vi "Dummy functional data generator.vi"() -> ()   [LabVIEW 2020]
uses:
  User Interface/Visualisation/Functional Imaging Viewer/SubVIs/Experiment header interface/Typedefs/Header file interface module functions enum.ctl
  Typedefs/Imaging Protocols enum.ctl
  Typedefs/Logging queue element.ctl
  Typedefs/Frame Size.ctl
  Typedefs/Acquired points count.ctl
panel:
  in  "Array":T1[](array[typedef]) {"Ref Dwell time (us)" format="%#.6g"; "Frame Size" items=["100X100"=100, "128X128"=128, "200X200"=200, "256X256"=256, "512X512"=512, "1024x1024"=1024, "2048x2048"=2048]; "Dwell time (us)" format="%#.6g"}
  out "error out":errorcluster
  in  "File path of existing dataset":path=path "C:/Functional Imaging Code/Data_Dummy generated -1POI 1Mscn"
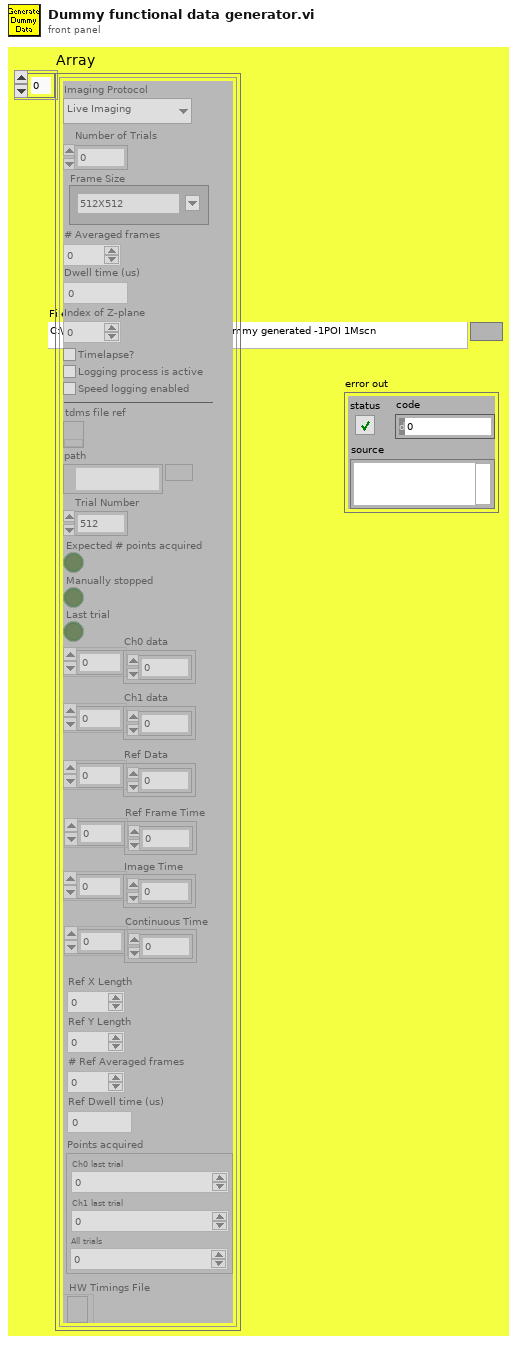
[diagram p1: front panel]
types:
  T1 = typedef "Logging queue element.ctl" = cluster{"Imaging Protocol":T2, "Number of Trials":u16, "Frame Size":T3, "# Averaged frames":u16, "Dwell time (us)":dbl, "Index of Z-plane":i32, "Timelapse?":bool, "Logging process is active":bool, "Speed logging enabled":bool, "tdms file ref":refnum<k34>, "path":path, "Trial Number":i32, "Expected # points acquired":bool, "Manually stopped":bool, "Last trial":bool, "Ch0 data":u32[], "Ch1 data":u32[], "Ref Data":u32[], "Ref Frame Time":u64[], "Image Time":u64[], "Continuous Time":u64[], "Ref X Length":u16, "Ref Y Length":u16, "# Ref Averaged frames":u16, "Ref Dwell time (us)":dbl, "Points acquired":T4, "HW Timings File":refnum<file>}
  T2 = typedef "Imaging Protocols enum.ctl" = enum16{"AOL Z-Stack", "Motor Z Stack", "Functional Acquisition", "Single Plane Acquisition", "Volume Acquisition", "Live Imaging", "Live Plane Imaging", "Live Volume Imaging"}
  T3 = typedef "Frame Size.ctl" = u16
  T4 = typedef "Acquired points count.ctl" = cluster{"Ch0 last trial":u64, "Ch1 last trial":u64, "All trials":u64}
  T5 = typedef "Header file interface module functions enum.ctl" = enum16{"Load experiment header file", "Save experiment header file", "Clear stored values", "Read stored values", "Update specific value in memory", "Update values in memory"}
  T6 = typedef "Header parameters cluster-ALL.ctl" = cluster{"LOGIN":T7, "GLOBAL PARAMETERS":T8, "IMAGING MODES":T10, "TIME SERIES":T11, "MOTOR Z-STACK ":T13, "AOL Z-STACK":T14, "FUNCTIONAL IMAGING":T15, "VOLUME IMAGING":T15, "MOVEMENT CORRECTION":T19, "CALIBRATION":T21, "STATISTICS":T22, "BIOLOGY INFORMATION":T23, "Calibration Data":T24}
  T7 = typedef "Header params -Login.ctl" = cluster{"User":string, "Profile":string, "Software Version":string, "Experiment Date Time":timestamp}
  T8 = typedef "Header params-Global Parameters.ctl" = cluster{"MicroscopeID":string, "Microscope Type":string, "Objective":string, "Field of View (um)":dbl, "Fill time (us)":dbl, "Experiment Type":T9, "Stimuli Trigger":bool, "Speed Logging":bool}
  T9 = typedef "Experiment Type.ctl" = enum16{"In vivo", "In vitro", "Testing", "Calibration", "Other"}
  T10 = typedef "Header params-Imaging Modes.ctl" = cluster{"Time Series":bool, "Motor Zstack":bool, "AOL Zstack":bool, "Functional Imaging":bool, "Volume Imaging":bool}
  T11 = typedef "Header params-Time Series.ctl" = cluster{"Basic Image meta data":T12, "AOL z":dbl}
  T12 = typedef "Header params-Basic image meta data.ctl" = cluster{"Wavelength (nm)":dbl, "# averaged frames":dbl, "laser power (%)":dbl, "Pockels":dbl, "pixel dwell time (us)":dbl, "pmt 1":dbl, "pmt 2":dbl, "back apperture":dbl, "zoom":dbl, "field of view":dbl, "Frame Size":T3, "AOL x centre":dbl, "AOL y centre":dbl, "Stage x position":dbl, "Stage y position":dbl, "Stage z position":dbl}
  T13 = typedef "Header params-Motor Z-stack.ctl" = cluster{"Hdr Basic Image meta data":T12, "Z Start":dbl, "Z Stop":dbl, "No of Planes":i32, "Laser Power (%) at Z Start":dbl, "Laser Power (%) at Z Stop":dbl}
  T14 = typedef "Header params-AOL Z-stack.ctl" = cluster{"Hdr Basic Image meta data":T12, "Z Start":dbl, "Z Stop":dbl, "No of Planes":i32, "Laser Power (%) at Z Start":dbl, "Laser Power (%) at Z Stop":dbl}
  T15 = typedef "Header params-Functional Imaging.ctl" = cluster{"Functional Mode":T16, "Variable Length":bool, "Variable Resolution":bool, "Pockels Modulation":bool, "Stimuli Trigger":bool, "Cool down enabled":bool, "AOL Mode":T17, "Plane Mode":T18, "Miniscan Dwell time per pixel (us)":dbl, "poi dwell time":dbl, "Number of trials":dbl, "Number of cycles":dbl, "Number of pois":dbl, "Number of miniscans":dbl, "Number of pixels in miniscan":dbl, "Rectangle ROI length":dbl, "Rectangle ROI height":dbl, "Frame rate (fps)":dbl, "Acquisition Length":dbl, "video length (sec)":dbl, "Stimuli delay (sec)":dbl, "Cool down time (sec)":dbl, "Basic Image meta data":T12, "Z Start (um)":dbl, "Z Stop (um)":dbl}
  T16 = typedef "Functional Mode.ctl" = enum16{"Point", "Line", "Patch", "Plane", "Volume"}
  T17 = typedef "AOL modes.ctl" = enum16{"Raster", "Structural", "Pointing", "Mini Scan", "Alignment"}
  T18 = typedef "Plane Mode.ctl" = u16
  T19 = typedef "Header params-Movement correction.ctl" = cluster{"Movement Correction":bool, "Axial Reference":bool, "Reference Source":T20, "Full Frame Size":dbl, "Reference Field of View":dbl, "Reference Zoom":dbl, "Reference dwell time (us)":dbl, "Reference X Pixels":dbl, "Reference Y Pixels":dbl, "Number of Z lines":dbl, "Size of Z pixels":dbl, "Axial Pixels":dbl, "Ignore Z lines":dbl, "Reference Scan Cycles":dbl, "Reference Threshold XY":dbl, "Reference Threshold Z":dbl, "Reference Average XY":dbl, "Reference Average Z":dbl, "Proportional Scale":dbl, "Integral Scale":dbl, "Proportional Scale Z":dbl, "Integral Scale Z":dbl, "Diff Threshold":dbl, "Diff Threshold Z":dbl, "Sliding Average":bool, "Reference count reset enabled":bool, "Scan Interval (ms)":dbl, "Ref Plot Refresh Rate (ms)":dbl}
  T20 = typedef "Reference source.ctl" = enum16{"Green channel", "Red channel"}
  T21 = typedef "Header params-Calibration Setup.ctl" = cluster{"Pockels Calibration File":path, "Calibration_ini file":path, "Setup_ini file":path}
  T22 = typedef "Header params-statistics.ctl" = cluster{"Z-stack duration (sec)":dbl, "Number of acquired data-points":dbl, "Acquisition time (ms)":dbl, "Number of acquired frames":dbl, "Intertrial times":dbl[]}
  T23 = typedef "Biology Information.ctl" = cluster{"Animal Code or Name":string, "Animal DoB":string, "Animal Age":string, "Animal Sex":string, "Animal Weight":string, "Date of Injection":string, "Date of Implant":string, "Site of Injection":string, "Animal Ear Notch":string, "AAV constructs":string, "Genetic background":string, "Optical reporter":string, "Region of brain imaged":string, "Other \ncomments":string}
  T24 = typedef "Header params-calibration data.ctl" = cluster{"Objective Name":string, "Calibration Wavelength":dbl, "Sum X":dbl, "Sum Y":dbl, "Diff X":dbl, "Diff Y":dbl, "Distortion Correction":dbl, " Z norm to um Scaling":dbl, " X norm to um Scaling":dbl}
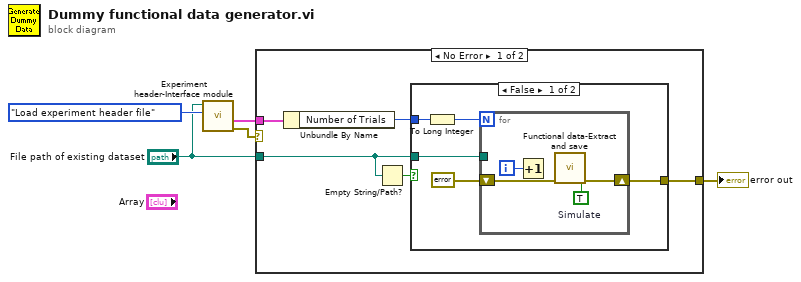
[diagram p0: block diagram]
diagram:
  n1 = call "Experiment header-Interface module.vi"("Function"=Header_file_interface_module_functions_enum."Load experiment header file", "Experiment data folder path"="File path of existing dataset") -> ("error out"=w1:errorcluster, "All header parameters out"=w2:T6)  [unwired: 8 in]
  n2 = case shown="No Error" w1 {
    tunnel: [w10 _] -> w5
    tunnel: "File path of existing dataset" -> [w7 _]
    tunnel: w2 -> [w6 _]
    frame No Error {
      n3 = Unbundle By Name(w6) -> ("Number of Trials"=w8:u16)
      n4 = Empty String/Path?(string/path=w7) -> (empty?=w9:bool)
      n5 = case shown="False" w9 {
        tunnel: w7 -> [w15 _]
        tunnel: w8 -> [w13 _]
        tunnel: [w12 _] -> w10
        frame False {
          n6 = To Long Integer(number=w13) -> (32bit integer=w11:i32)
          n7 = for {
            N: w11 -> [_]
            tunnel: w15 -> [_]
            shift-right: [w19] -> w12
            shift-left: errorcluster {"status"=FALSE, "code"=0, "source"=""} ("error out") -> [w18]
            i -> [w17]
            w16 = TRUE  # Simulate
            n8 = Increment(x=w17) -> ()  [unwired: 1 out]
            n9 = call "Functional data-Extract and save.vi"("Simulate"=w16, "error in (no error)"=w18) -> ("error out"=w19:errorcluster)  [unwired: 8 in, 1 out]
          }
        }
        frame True {
        }
      }
    }
    frame Error {
    }
  }
  "error out" <- w5
